vi "FinalProject.vi"() -> ()   [LabVIEW 2020]
panel:
  out "No Motion Detected":bool
  out "Motion Detected":bool
  in  "Object":bool
  in  "Motion":bool
  in  "VISA resource name":refnum<visa-resource-name>
  in  "Table Control":string[][](table)
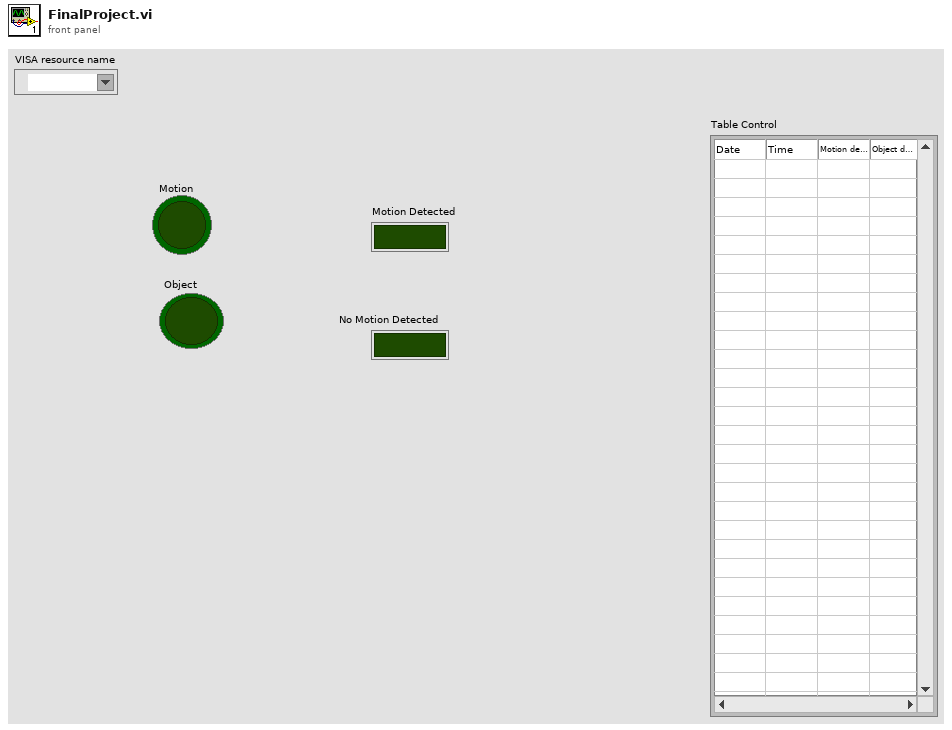
[diagram p1: front panel]
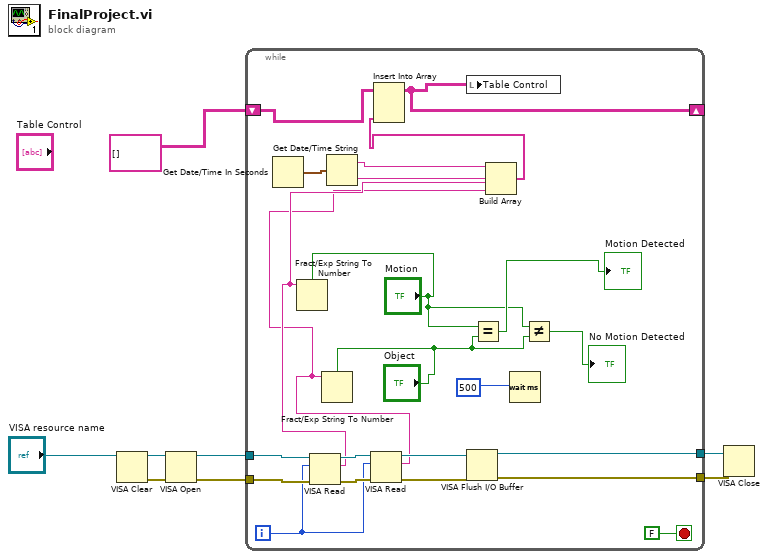
[diagram p0: block diagram]
diagram:
  n1 = VISA Clear(VISA resource name="VISA resource name") -> (VISA resource name out=w7:refnum<visa-resource-name>, error out=w8:errorcluster)  [unwired: 1 in]
  n2 = VISA Open(error in (no error)=w8, VISA resource name=w7) -> (VISA resource name=w5:refnum<visa-resource-name>, error out=w6:errorcluster)  [unwired: 3 in]
  n3 = while {
    tunnel: w6 -> [w27]
    tunnel: w5 -> [w31]
    tunnel: [w28] -> w4
    tunnel: [w24] -> w3
    shift-right: [w20] -> _
    shift-left: string[][] [] -> [w21]
    i -> [w23]
    stop <- FALSE stop-if-true
    n4 = Get Date/Time In Seconds() -> (seconds since 1Jan1904=w19:timestamp)
    n5 = VISA Read(VISA resource name=w31, byte count=w23, error in (no error)=w27) -> (VISA resource name out=w30:refnum<visa-resource-name>, read buffer=w16:string, error out=w26:errorcluster)  [unwired: 1 out]
    n6 = Fract/Exp String To Number(use system decimal point (T)="Motion", string=w16) -> ()  [unwired: 2 in, 2 out]
    n7 = Get Date/Time String(seconds (now)=w19) -> (date string=w18:string, time string=w17:string)  [unwired: 2 in]
    n8 = VISA Read(VISA resource name=w30, byte count=w23, error in (no error)=w26) -> (VISA resource name out=w29:refnum<visa-resource-name>, read buffer=w11:string, error out=w25:errorcluster)  [unwired: 1 out]
    n9 = Fract/Exp String To Number(use system decimal point (T)="Object", string=w11) -> ()  [unwired: 2 in, 2 out]
    n10 = VISA Flush I/O Buffer(VISA resource name=w29, error in (no error)=w25) -> (VISA resource name out=w28:refnum<visa-resource-name>, error out=w24:errorcluster)  [unwired: 1 in]
    n11 = Equal?(x="Motion", y="Object") -> (x = y?=→"Motion Detected":bool)
    n12 = Build Array(w18, w17, w16, w11) -> (w15:string[])
    n13 = Insert Into Array(array=w21, new element=w15) -> (w20:string[][])  [unwired: 2 in]
    n14 = local write "Table Control"(w20) -> ()
    n15 = Wait (ms)(milliseconds to wait=u32 500) -> ()  [unwired: 1 out]
    n16 = Not Equal?(x="Motion", y="Object") -> (x != y?=→"No Motion Detected":bool)
  }
  n17 = VISA Close(VISA resource name=w4, error in (no error)=w3) -> ()  [unwired: 1 out]
